vi "RoutePlaner.vi"(7 "Origin In":cluster{"X":sgl, "Y":sgl, "Z":sgl}, 9 "Pixel Size(mm)":dbl=1.0, 10 "Y distance(mm)":dbl=10.0, 11 "X distance (mm)":dbl=10.0) -> (1 "TotalDistance (mm)":dbl, 2 "PtArray":cluster{"x":dbl, "y":dbl, "z":dbl}[](array[cluster]), 3 "output cluster":cluster{"X":dbl[], "Y":dbl[], "Z":dbl[]})   [LabVIEW 2024]
panel:
  out "size(s)":i32
  out "XY Graph":cluster{dbl[], dbl[]}(graph)
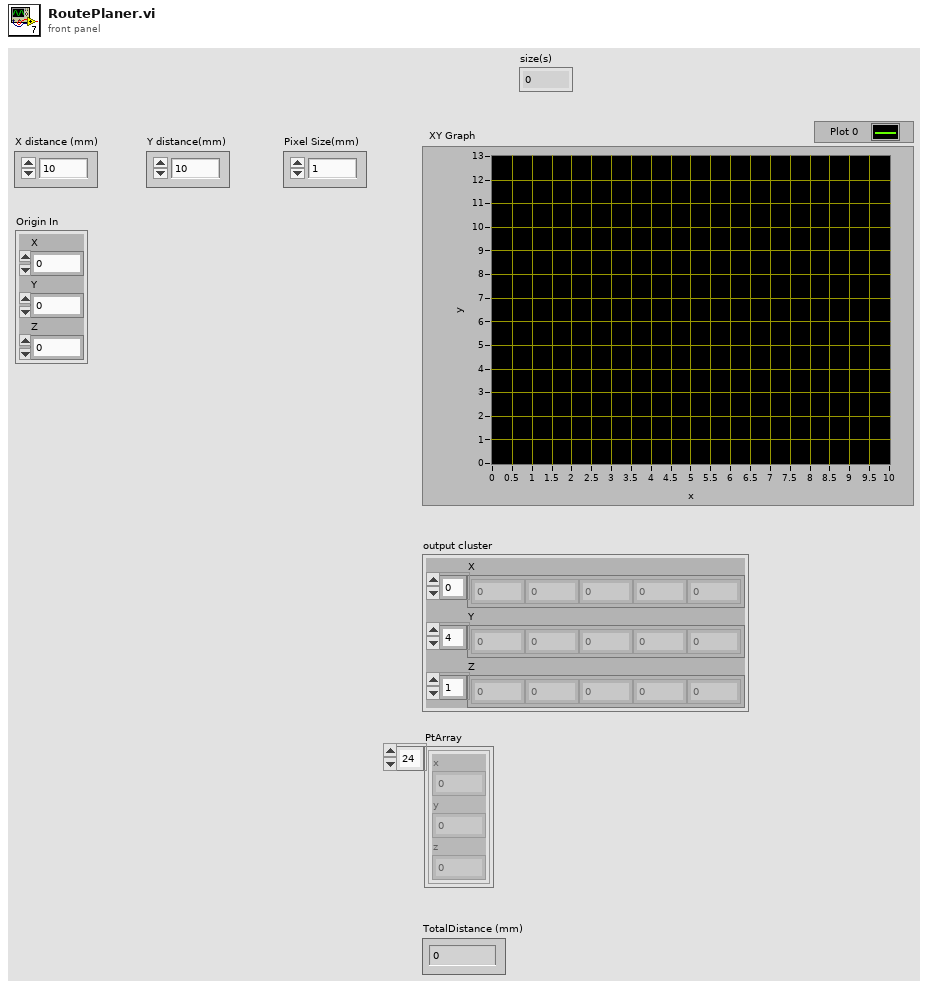
[diagram p1: front panel]
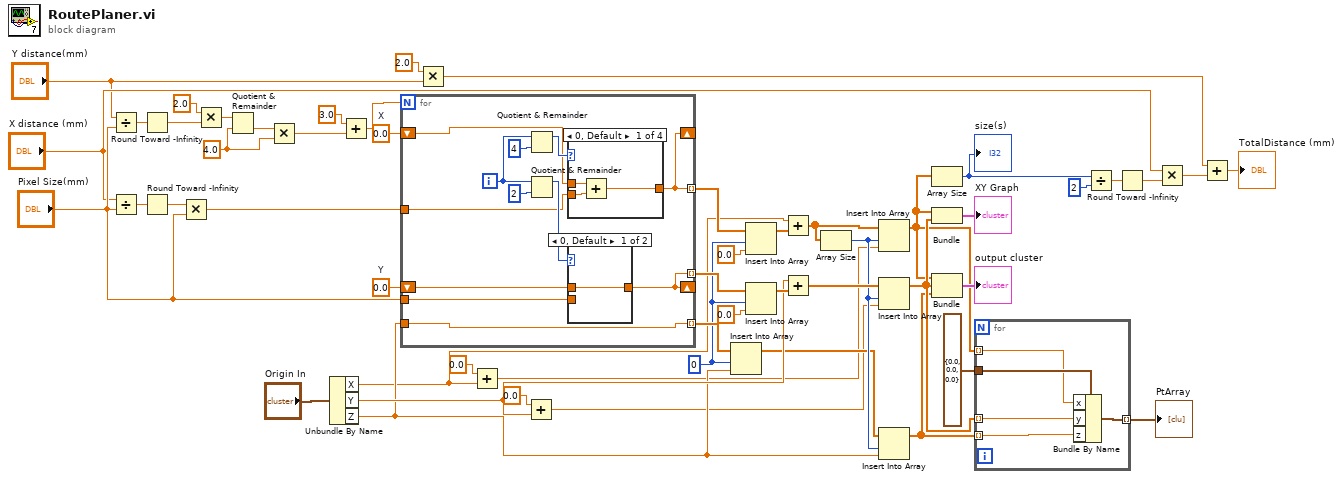
[diagram p0: block diagram]
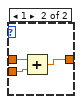
[diagram p2: hidden frame]
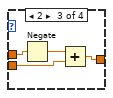
[diagram p4: hidden frame]
diagram:
  w27 = 4.0 ("y")
  w35 = 0 ("index")
  w48 = 0.0  # X
  w49 = 0.0  # Y
  n1 = Divide(x="Y distance(mm)", y="Pixel Size(mm)") -> (x/y=w51:dbl)
  n2 = Divide(x="X distance (mm)", y="Pixel Size(mm)") -> (x/y=w52:dbl)
  n3 = Round Toward -Infinity(1:w51) -> (0:w13:dbl)
  n4 = Round Toward -Infinity(1:w52) -> (0:w50:dbl)
  n5 = Multiply(x=w50, y="Pixel Size(mm)") -> (x*y=w47:dbl)
  n6 = Multiply(x=2.0, y=w13) -> (x*y=w29:dbl)
  n7 = Quotient & Remainder(x=w29, y=w27) -> (floor(x/y)=w28:dbl)  [unwired: 1 out]
  n8 = Multiply(x=w28, y=w27) -> (x*y=w26:dbl)
  n9 = Unbundle By Name("Origin In") -> ("X"=w23:sgl, "Y"=w32:sgl, "Z"=w30:sgl)
  n10 = Add(x=3.0, y=w26) -> (x+y=w24:dbl)
  n11 = for {
    N: w24 -> [_]
    tunnel: "Pixel Size(mm)" -> [w61]
    tunnel: [w60] -> w44 mode=indexing
    tunnel: [w58] -> w33 mode=indexing
    shift-right: [w60] -> _
    shift-left: w49 -> [w62]
    shift-right: [w58] -> _
    shift-left: w48 -> [w53]
    tunnel: w47 -> [w59]
    tunnel: w30 -> [w54]
    tunnel: [w54] -> w38 mode=indexing
    i -> [w57]
    n12 = Quotient & Remainder(x=w57, y=4) -> (x-y*floor(x/y)=w55:i32)  [unwired: 1 out]
    n13 = Quotient & Remainder(x=w57, y=2) -> (x-y*floor(x/y)=w63:i32)  [unwired: 1 out]
    n14 = case shown="0, Default" w55 {
      tunnel: [w71 w72 w76 w77] -> w58
      tunnel: w53 -> [w70 w72 w75 w77]
      tunnel: w59 -> [w69 _ w74 _]
      frame 0, Default {
        n15 = Add(x=w70, y=w69) -> (x+y=w71:dbl)
      }
      frame 1 {
      }
      frame 2 {
        n16 = Negate(x=w75) -> (-x=w73:dbl)
        n17 = Add(x=w73, y=w74) -> (x+y=w76:dbl)
      }
      frame 3 {
      }
    }
    n18 = case shown="0, Default" w63 {
      tunnel: w62 -> [w65 w67]
      tunnel: [w65 w68] -> w60
      tunnel: w61 -> [_ w66]
      frame 0, Default {
      }
      frame 1 {
        n19 = Add(x=w67, y=w66) -> (x+y=w68:dbl)
      }
    }
  }
  n20 = Multiply(x=2.0, y="Y distance(mm)") -> (x*y=w3:dbl)
  n21 = Add(x=sgl 0.0, y=w23) -> (x+y=w22:sgl)
  n22 = Add(x=sgl 0.0, y=w32) -> (x+y=w20:sgl)
  n23 = Insert Into Array(array=w38, index=w35, new element=w30) -> (w31:sgl[])
  n24 = Insert Into Array(array=w33, index=w35, new element=0.0 ("new element/subarray")) -> (w46:dbl[])
  n25 = Insert Into Array(array=w44, index=w35, new element=0.0 ("new element/subarray")) -> (w43:dbl[])
  n26 = Add(x=w23, y=w46) -> (x+y=w36:dbl[])
  n27 = Add(x=w32, y=w43) -> (x+y=w40:dbl[])
  n28 = Array Size(array=w36) -> (size(s)=w34:i32)
  n29 = Insert Into Array(array=w36, index=w34, new element=w22) -> (w11:dbl[])
  n30 = Insert Into Array(array=w40, index=w34, new element=w20) -> (w17:dbl[])
  n31 = Insert Into Array(array=w31, index=w34, new element=w30) -> (w16:sgl[])
  n32 = Array Size(array=w11) -> (size(s)=w10:i32)
  "size(s)" <- w10
  n33 = Bundle(w11, w17) -> (→"XY Graph":cluster{dbl[], dbl[]})  [unwired: 1 in]
  n34 = Bundle(w11, w17, w16) -> (→"output cluster":cluster{dbl[], dbl[], sgl[]})  [unwired: 1 in]
  n35 = for {
    tunnel: cluster{"x":dbl, "y":dbl, "z":dbl} {"x"=0.0, "y"=0.0, "z"=0.0} -> [w82]
    tunnel: w11 -> [w81] mode=indexing
    tunnel: w17 -> [w80] mode=indexing
    tunnel: w16 -> [w79] mode=indexing
    tunnel: [w78] -> w15 mode=indexing
    n36 = Bundle By Name(cluster=w82, "x"=w81, "y"=w80, "z"=w79) -> (w78:cluster{"x":dbl, "y":dbl, "z":dbl})
  }
  "PtArray" <- w15
  n37 = Divide(x=w10, y=2) -> (x/y=w8:dbl)
  n38 = Round Toward -Infinity(1:w8) -> (0:w1:dbl)
  n39 = Multiply(x="X distance (mm)", y=w1) -> (x*y=w6:dbl)
  n40 = Add(x=w3, y=w6) -> (x+y=→"TotalDistance (mm)":dbl)
